vi "Keithley 6517A Triggering Control.vi"(2 "Trigger Control (Reset Triggering:0)":u16(ring) items=["Reset Triggering", "Initiate One Trigger Cycle", "Initiate Continuous Triggering", "Send Bus Trigger"], 3 "error in":T1, 5 "GPIB address":string="27") -> (0 "error out":T1)   [LabVIEW 2013]
doc: "This VI is used to control triggering in the 6517A.\n\nParameters:\n\nTrigger Control:\n0 = Reset Triggering\n1 = Initiate One Trigger Cycle\n2 = Initiate Continuous Triggering\n3 = Send Bus Trigger"
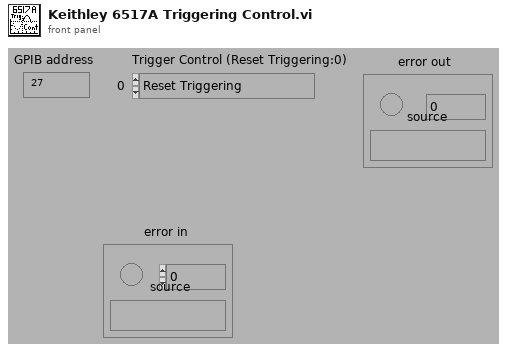
[diagram p1: front panel]
types:
  T1 = cluster{"error":bool, "code":i32, "source":string}
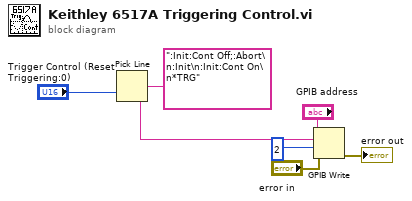
[diagram p0: block diagram]
diagram:
  n1 = Pick Line(multi-line string=":Init:Cont Off;:Abort\n:Init\n:Init:Cont On\n*TRG", line index="Trigger Control (Reset Triggering:0)") -> (output string=w1:string)  [unwired: 1 in]
  n2 = GPIB Write(0:"GPIB address", 1:w1, 2:2, 3:"error in") -> (6:→"error out":errorcluster)  [unwired: 1 in, 1 out]
